vi "Handle Error.vi"(8 "error in (no error)":errorcluster, 11 "UI ActorTop in":refnum<class "CheckPasswordUI.lvclass">) -> (0 "error out":errorcluster, 2 "stop actor?":bool=TRUE, 3 "UI ActorTop out":refnum<class "CheckPasswordUI.lvclass">)   [LabVIEW 2021, in "CheckPasswordUI.lvclass"]
doc: "(<B>Filename</B>: Actor Framework.lvlib:Actor.lvclass:Handle Error.vi)\n\nDefines how the actor handles an error that occurred while processing a message. By default, this method does nothing except stop the actor."
uses:
  CheckPasswordUI.lvclass
  <userlib>/John_Lib/AbstractActorTemplate/AbstractActorTemplate/UIActorTop.lvclass
  CheckPasswordUI.lvclass/CheckPasswordUI.ctl
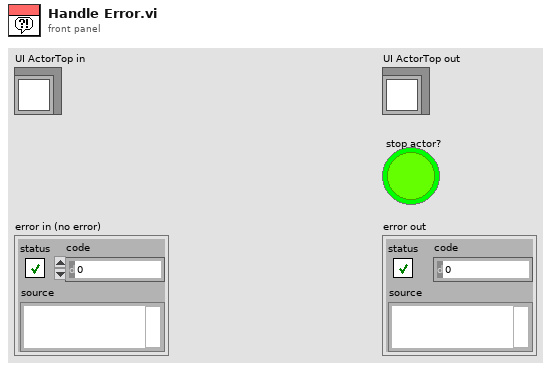
[diagram p1: front panel]
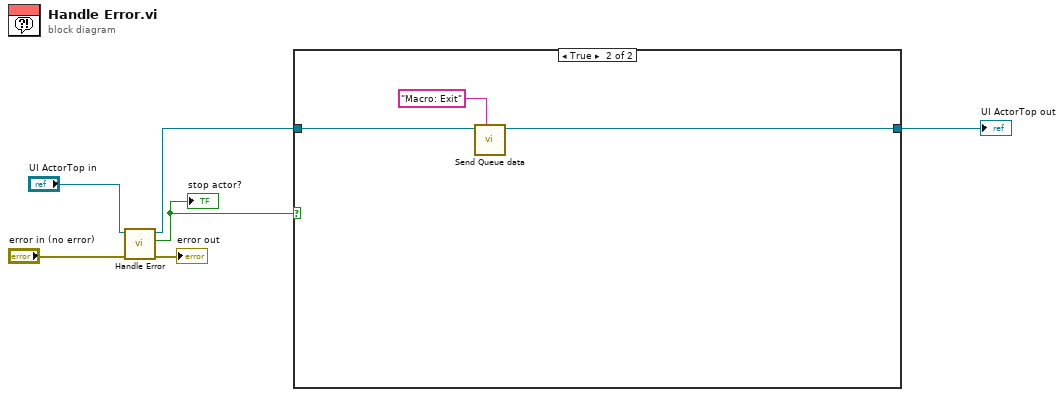
[diagram p0: block diagram]
diagram:
  n1 = call-parent "Handle Error.vi"("error in (no error)"="error in (no error)", "UI ActorTop in"="UI ActorTop in") -> ("error out"=→"error out":errorcluster, "stop actor?"=w3:bool, "UI ActorTop out"=w2:refnum<class "CheckPasswordUI.lvclass">)  [unwired: 7 in]
  "stop actor?" <- w3
  n2 = case shown="True" w3 {
    tunnel: w2 -> [w7 w9]
    tunnel: [w7 w10] -> w1
    frame False {
    }
    frame True {
      n3 = call "Send Queue data.vi"("Elements in Front"="Macro: Exit", "CheckPasswordUI in"=w9) -> ("CheckPasswordUI out"=w10:refnum<class "CheckPasswordUI.lvclass">)  [unwired: 8 in, 1 out]
    }
  }
  "UI ActorTop out" <- w1
